vi "Test Pixy2 Functionality.vi"() -> ()   [LabVIEW 2018]
uses:
  source/library/Types/Intersection.ctl
  source/library/Types/Vector.ctl
  <vilib>/Rock Robotics/SystemInterfaces/i2clib/i2c_bus.ctl
  source/library/Interface/Pixy Com.lvclass
  source/deviceSupport/FRC/I2C/RoboRIO I2C.lvclass
  source/library/Pixy2.lvlib
  <vilib>/Rock Robotics/SystemInterfaces/spilib/spi_bus.ctl
  source/deviceSupport/FRC/SPI/RoboRIO SPI.lvclass
  source/deviceSupport/FRC/UART/RoboRIO UART.lvclass
  <vilib>/Rock Robotics/WPI/SerialPort/WPI_SerialPort.ctl
panel:
  out "fps":u32
  out "vectors":T1[](array[typedef])
  out "intersections":T2[](array[typedef])
  out "view":picture
  in  "Stop Button":bool
  in  "message":T3(tab)
  in  "color":cluster{"r":u8, "g":u8, "b":u8}
  in  "lamp enable":cluster{"upper":bool, "lower":bool}
  in  "signature map":u8=255 format="%.0x"
  in  "max blocks":u8=255
  in  "features":enum16{"Main Features", "All Features"}(ring)
  in  "feature map":u8=7 format="%.0x"
  in  "mode":u8 format="%.0x"
  in  "vector":u8
  out "Color":u32(colorbox)
  in  "saturate?":bool
  in  "y":u16 max=207
  in  "x":u16 max=315
  in  "brightness":u8
  out "error out":errorcluster
  in  "send":bool
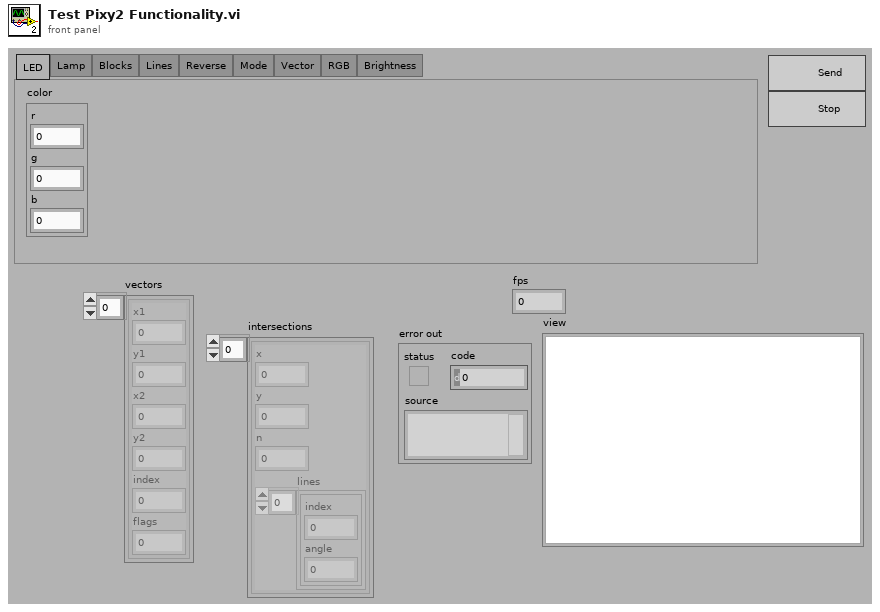
[diagram p1: front panel]
types:
  T1 = typedef "Pixy2.lvlib/Vector.ctl" = cluster{"x1":u8, "y1":u8, "x2":u8, "y2":u8, "index":u8, "flags":u8}
  T2 = typedef "Pixy2.lvlib/Intersection.ctl" = cluster{"x":u8, "y":u8, "n":u8, "lines":cluster{"index":u8, "angle":i16}[]}
  T3 = enum32{"LED", "Lamp", "Blocks", "Lines", "Reverse", "Mode", "Vector", "RGB", "Brightness"}
  T4 = typedef "i2c_bus.ctl" = enum16{"I2C On-Board", "I2C MXP", "Invalid"}
  T5 = typedef "spi_bus.ctl" = enum16{"SPI On-Board, CS0", "SPI On-Board, CS1", "SPI On-Board, CS2", "SPI On-Board, CS3", "SPI MXP", "Invalid"}
  T6 = typedef "WPI_SerialPort.ctl" = enum16{"Onboard RS-232", "MXP TTL", "USB 1", "USB 2"}
  T7 = typedef "Pixy2.lvlib/Block.ctl" = cluster{"signature":u16, "x":u16, "y":u16, "width":u16, "height":u16, "angle":i16, "index":u8, "age":u8}
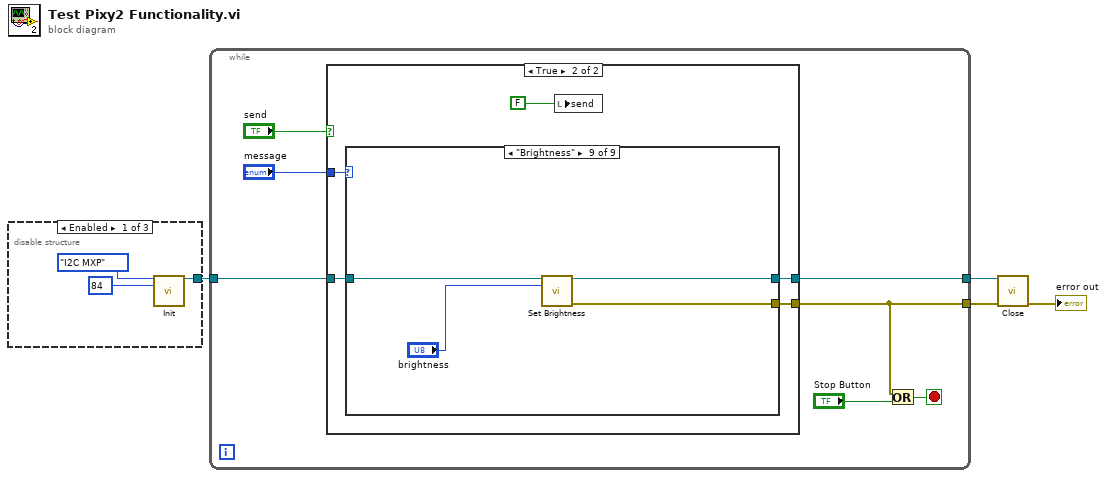
[diagram p0: block diagram]
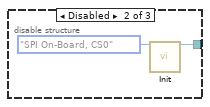
[diagram p2: hidden frame]
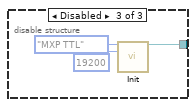
[diagram p3: hidden frame]
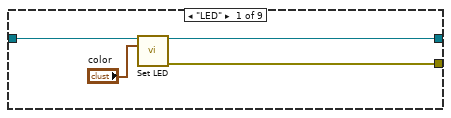
[diagram p5: hidden frame]
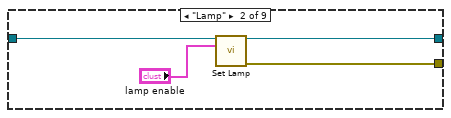
[diagram p6: hidden frame]
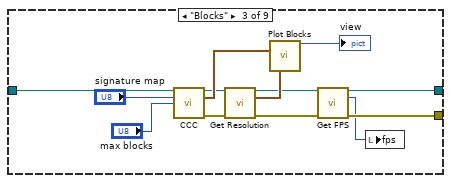
[diagram p7: hidden frame]
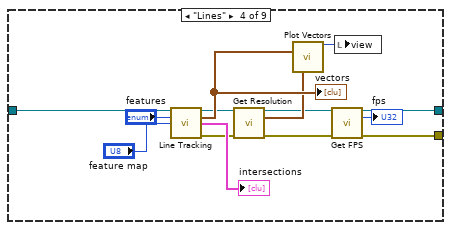
[diagram p8: hidden frame]
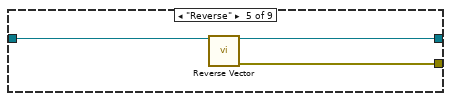
[diagram p9: hidden frame]
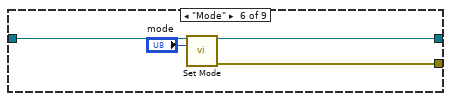
[diagram p10: hidden frame]
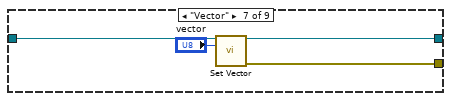
[diagram p11: hidden frame]
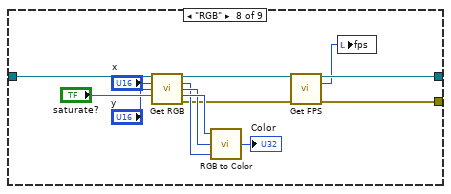
[diagram p12: hidden frame]
diagram:
  n1 = disable-structure shown="Enabled" {
    disable-tunnel: [w7 w9 w12] -> w4
    frame Enabled {
      n2 = call "Init.vi"("I2C bus"=i2c_bus."I2C MXP" ("I2C Bus"), "device address"=u8 84 ("Device Address")) -> ("comm interface out"=w7:refnum<class "Pixy Com.lvclass">)  [unwired: 12 in, 1 out]
    }
    frame Disabled {
      n3 = call "Init.vi"("SPI Bus"=spi_bus."SPI On-Board, CS0") -> ("comm interface out"=w9:refnum<class "Pixy Com.lvclass">)  [unwired: 13 in, 1 out]
    }
    frame Disabled {
      n4 = call "Init.vi"("serial port"=WPI_SerialPort."MXP TTL", "baud rate"=u32 19200) -> ("comm interface out"=w12:refnum<class "Pixy Com.lvclass">)  [unwired: 12 in, 1 out]
    }
  }
  n5 = while {
    tunnel: w4 -> [w18]
    tunnel: [w16] -> w3
    tunnel: [w17] -> w2
    stop <- w15 stop-if-true
    n6 = case shown="True" "send" {
      tunnel: w18 -> [w20 w24]
      tunnel: [_ w22] -> w16
      tunnel: [w20 w23] -> w17
      tunnel: "message" -> [_ w21]
      frame False {
      }
      frame True {
        n7 = case shown="\"Brightness\"" w21 {
          tunnel: w24 -> [w29 w33 w46 w60 w63 w67 w71 w84 w87]
          tunnel: [w28 w32 w35 w49 w62 w66 w70 w73 w86] -> w23
          tunnel: [w27 w30 w36 w48 w61 w65 w69 w75 w85] -> w22
          frame "LED" {
            n8 = call "Set LED.vi"("comm interface in"=w29, "color"="color") -> ("comm interface out"=w28:refnum<class "Pixy Com.lvclass">, "error out"=w27:errorcluster)  [unwired: 12 in]
          }
          frame "Lamp" {
            n9 = call "Set Lamp.vi"("comm interface in"=w33, "lamp enable"="lamp enable") -> ("comm interface out"=w32:refnum<class "Pixy Com.lvclass">, "error out"=w30:errorcluster)  [unwired: 12 in]
          }
          frame "Blocks" {
            n10 = call "CCC.vi"("comm interface in"=w46, "signature map"="signature map", "max blocks"="max blocks") -> ("comm interface out"=w41:refnum<class "Pixy Com.lvclass">, "blocks"=w43:T7[], "error out"=w40:errorcluster)  [unwired: 10 in]
            n11 = call "Get Resolution.vi"("comm interface in"=w41, "error in"=w40) -> ("comm interface out"=w38:refnum<class "Pixy Com.lvclass">, "resolution"=w39:cluster{"width":u16, "height":u16}, "error out"=w37:errorcluster)  [unwired: 11 in]
            n12 = call "Plot Blocks.vi"("blocks"=w43, "pixy resolution"=w39) -> ("picture out"=→"view":picture)  [unwired: 13 in]
            n13 = call "Get FPS.vi"("comm interface in"=w38, "error in"=w37) -> ("comm interface out"=w35:refnum<class "Pixy Com.lvclass">, "fps"=w34:u32, "error out"=w36:errorcluster)  [unwired: 11 in]
            n14 = local write "fps"(w34) -> ()
          }
          frame "Lines" {
            n15 = call "Line Tracking.vi"("comm interface in"=w60, "features"="features", "feature map"="feature map") -> ("comm interface out"=w54:refnum<class "Pixy Com.lvclass">, "vectors"=w57:T1[], "intersections"=→"intersections":T2[], "error out"=w53:errorcluster)  [unwired: 8 in, 1 out]
            "vectors" <- w57
            n16 = call "Get Resolution.vi"("comm interface in"=w54, "error in"=w53) -> ("comm interface out"=w51:refnum<class "Pixy Com.lvclass">, "resolution"=w52:cluster{"width":u16, "height":u16}, "error out"=w50:errorcluster)  [unwired: 11 in]
            n17 = call "Plot Vectors.vi"("vectors"=w57, "pixy resolution"=w52) -> ("picture out"=w56:picture)  [unwired: 13 in]
            n18 = call "Get FPS.vi"("comm interface in"=w51, "error in"=w50) -> ("comm interface out"=w49:refnum<class "Pixy Com.lvclass">, "fps"=→"fps":u32, "error out"=w48:errorcluster)  [unwired: 11 in]
            n19 = local write "view"(w56) -> ()
          }
          frame "Reverse" {
            n20 = call "Reverse Vector.vi"("comm interface in"=w63) -> ("comm interface out"=w62:refnum<class "Pixy Com.lvclass">, "error out"=w61:errorcluster)  [unwired: 13 in]
          }
          frame "Mode" {
            n21 = call "Set Mode.vi"("comm interface in"=w67, "mode"="mode") -> ("comm interface out"=w66:refnum<class "Pixy Com.lvclass">, "error out"=w65:errorcluster)  [unwired: 12 in]
          }
          frame "Vector" {
            n22 = call "Set Vector.vi"("comm interface in"=w71, "vector"="vector") -> ("comm interface out"=w70:refnum<class "Pixy Com.lvclass">, "error out"=w69:errorcluster)  [unwired: 12 in]
          }
          frame "RGB" {
            n23 = call "Get RGB.vi"("comm interface in"=w84, "x"="x", "y"="y", "saturate?"="saturate?") -> ("comm interface out"=w74:refnum<class "Pixy Com.lvclass">, "blue"=w80:u8, "green"=w81:u8, "red"=w82:u8, "error out"=w76:errorcluster)  [unwired: 7 in]
            n24 = call <vilib>:"RGB to Color.vi"("B"=w80, "G"=w81, "R"=w82) -> ("Color"=→"Color":u32)
            n25 = call "Get FPS.vi"("comm interface in"=w74, "error in"=w76) -> ("comm interface out"=w73:refnum<class "Pixy Com.lvclass">, "fps"=w72:u32, "error out"=w75:errorcluster)  [unwired: 11 in]
            n26 = local write "fps"(w72) -> ()
          }
          frame "Brightness" {
            n27 = call "Set Brightness.vi"("comm interface in"=w87, "brightness"="brightness") -> ("comm interface out"=w86:refnum<class "Pixy Com.lvclass">, "error out"=w85:errorcluster)  [unwired: 12 in]
          }
        }
        n28 = local write "send"(FALSE ("send button")) -> ()
      }
    }
    n29 = Or(x=w16, y="Stop Button") -> (x .or. y?=w15:bool)
  }
  n30 = call-dynamic "Close.vi"("comm interface in"=w2, "error in"=w3) -> ("error out"=→"error out":errorcluster)  [unwired: 13 in]
